vi "pwm_out - 副本.vi"(0 "pwm info":T1={"sample mode"=10178, "initial delay"=0.0, "idle state"=10214, "counter"="Dev1/ctr0", "channel name"="pwm out", "low time"=0.01, "high time"=0.01, "units"=10364, "number of samples"=100} {"sample mode" items=["Finite Samples"=10178, "Continuous Samples"=10123, "Hardware Timed Single Point"=12522]; "idle state" items=["High"=10192, "Low"=10214]; "units" items=["Seconds"=10364, "From Custom Scale"=10065]}, 11 "error in":errorcluster caption="错误输入") -> (15 "error out":errorcluster caption="错误输出")   [LabVIEW 2013]
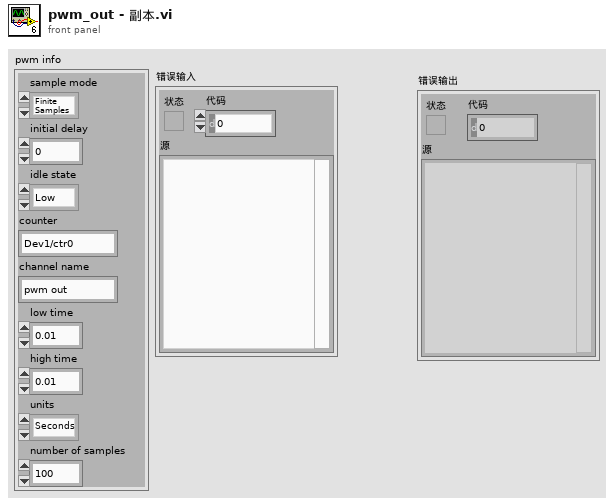
[diagram p1: front panel]
types:
  T1 = cluster{"sample mode":i32, "initial delay":dbl, "idle state":i32, "counter":string, "channel name":string, "low time":dbl, "high time":dbl, "units":i32, "number of samples":i32}
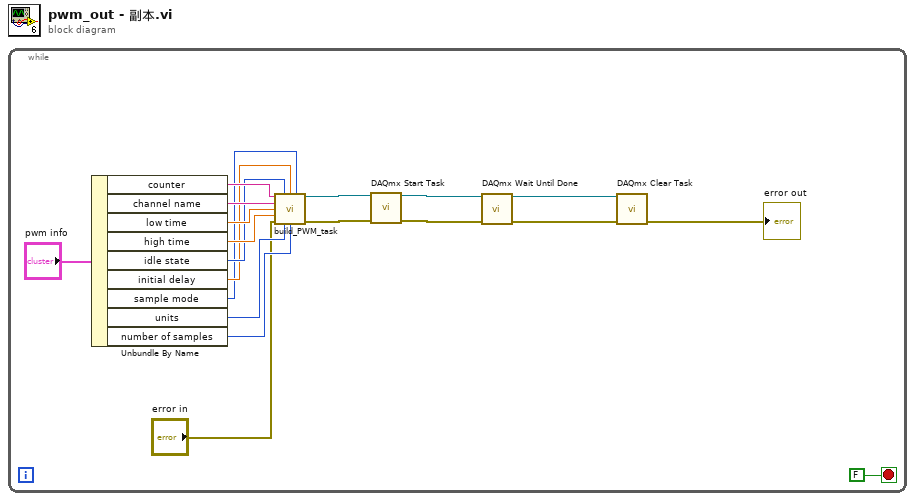
[diagram p0: block diagram]
diagram:
  n1 = while {
    stop <- FALSE stop-if-true
    n2 = Unbundle By Name("pwm info") -> ("counter"=w11:string, "channel name"=w10:string, "low time"=w9:dbl, "high time"=w8:dbl, "idle state"=w7:i32, "initial delay"=w6:dbl, "sample mode"=w5:i32, "units"=w4:i32, "number of samples"=w3:i32)
    n3 = call "build_PWM_task.vi"("counter"=w11, "idle state"=w7, "initial delay"=w6, "sample mode"=w5, "channel name"=w10, "low time"=w9, "high time"=w8, "error in"="error in", "units"=w4, "number of samples"=w3) -> ("task out"=w15:refnum<k21>, "error out"=w14:errorcluster)  [unwired: 4 in]
    n4 = call <vilib>:"DAQmx Start Task.vi"("task/channels in"=w15, "error in"=w14) -> ("task out"=w19:refnum<k21>, "error out"=w18:errorcluster)  [unwired: 12 in]
    n5 = call <vilib>:"DAQmx Wait Until Done.vi"("task/channels in"=w19, "error in"=w18) -> ("task out"=w16:refnum<k21>, "error out"=w17:errorcluster)  [unwired: 12 in]
    n6 = call <vilib>:"DAQmx Clear Task.vi"("task in"=w16, "error in"=w17) -> ("error out"=→"error out":errorcluster)  [unwired: 13 in]
  }
